vi "linear step ramp.vi"(0 "start":dbl, 7 "N ramps":i32, 11 "End":dbl) -> (4 "Array size":i32, 8 "Vakues array":dbl[](array[numeric]), 15 "Ramp Step":dbl)   [LabVIEW 2019]
doc: "Linear ramp using while loop \n\nJuan Gamez\n\nP3600"
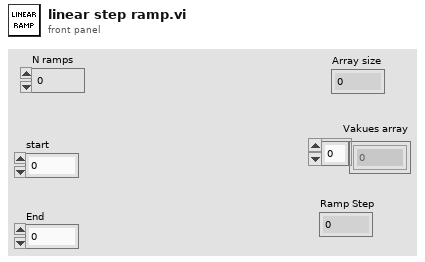
[diagram p1: front panel]
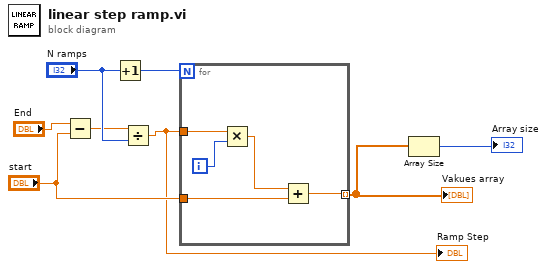
[diagram p0: block diagram]
diagram:
  n1 = Subtract(x="End", y="start") -> (x-y=w5:dbl)
  n2 = Increment(x="N ramps") -> (x+1=w8:i32)
  n3 = Divide(x=w5, y="N ramps") -> (x/y=w1:dbl)
  "Ramp Step" <- w1
  n4 = for {
    N: w8 -> [_]
    tunnel: w1 -> [w12]
    tunnel: "start" -> [w10]
    tunnel: [w9] -> w3 mode=indexing
    i -> [w13]
    n5 = Multiply(x=w12, y=w13) -> (x*y=w11:dbl)
    n6 = Add(x=w11, y=w10) -> (x+y=w9:dbl)
  }
  "Vakues array" <- w3
  n7 = Array Size(array=w3) -> (size(s)=→"Array size":i32)
